vi "CreateDigitalWaveform.vi"() -> (0 "digital waveform out":digitalwaveform(graph))   [LabVIEW 2018]
uses:
  <vilib>/Waveform/DWDTOps.llb/Digital Pattern Generator (Single Value).vi
  <vilib>/Waveform/DWDTOps.llb/DWDT Append Digital Samples.vi
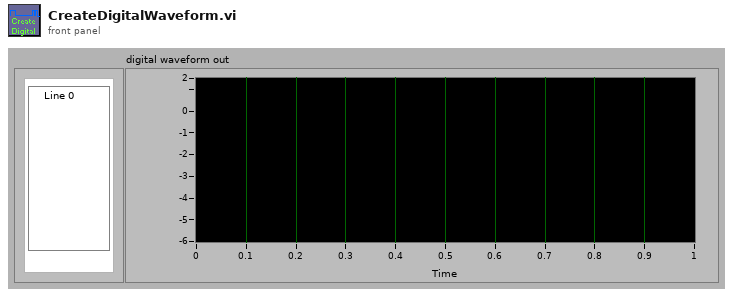
[diagram p1: front panel]
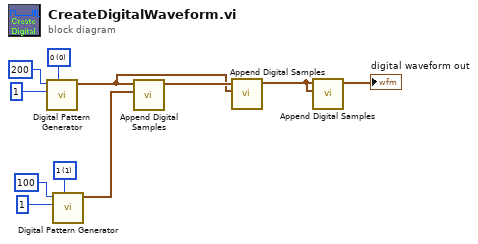
[diagram p0: block diagram]
diagram:
  w8 = u8 1 items=["0", "1", "Z", "L", "H", "X", "T", "V"] ("value")
  w7 = u8 0 items=["0", "1", "Z", "L", "H", "X", "T", "V"] ("value")
  n1 = call-poly <vilib>:"Digital Pattern Generator.vi"("value"=w7, "number of signals"=u32 1, "number of samples"=u32 200) -> ("digital waveform"=w1:digitalwaveform)  [unwired: 2 in, 6 out]
  n2 = call-poly <vilib>:"Digital Pattern Generator.vi"("value"=w8, "number of signals"=u32 1, "number of samples"=u32 100) -> ("digital waveform"=w11:digitalwaveform)  [unwired: 2 in, 6 out]
  n3 = call-poly <vilib>:"Append Digital Samples.vi"("digital waveform B"=w11, "digital waveform A"=w1) -> ("digital waveform out"=w2:digitalwaveform)  [unwired: 1 in, 8 out]
  n4 = call-poly <vilib>:"Append Digital Samples.vi"("digital waveform B"=w1, "digital waveform A"=w2) -> ("digital waveform out"=w4:digitalwaveform)  [unwired: 1 in, 8 out]
  n5 = call-poly <vilib>:"Append Digital Samples.vi"("digital waveform B"=w4, "digital waveform A"=w4) -> ("digital waveform out"=→"digital waveform out":digitalwaveform)  [unwired: 1 in, 8 out]
